vi "Convert cluster to array.vi"(8 "error in (no error)":errorcluster, 10 "cluster":variant) -> (0 "error out":errorcluster, 2 "array":variant[](array[variant]))   [LabVIEW 2023, in "uData.lvlib" / "uData.lvclass"]
doc: "Convert incoming cluster to array."
uses:
  uData.lvclass
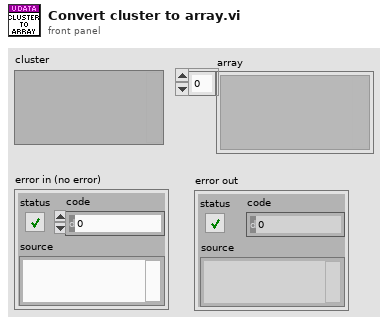
[diagram p1: front panel]
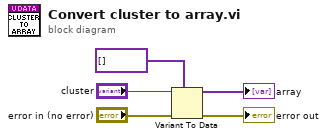
[diagram p0: block diagram]
diagram:
  n1 = Variant To Data(error in="error in (no error)", type=variant[] [] ("Array"), Variant="cluster") -> (data=→"array":variant[], error out=→"error out":errorcluster)
